vi "Copy.vi"(8 "error in (no error)":errorcluster, 10 "NT Base in":refnum<class "NT Base.lvclass">, 11 "NT Base in":refnum<class "NT Base.lvclass">) -> (0 "error out":errorcluster, 3 "NT Base out":refnum<class "NT Base.lvclass">)   [LabVIEW 2020, in "PV Access.lvlib" / "PV Data.lvlib" / "NT Base.lvclass"]
uses:
  NT Base.lvclass
  NT Base.lvclass/NT Base.ctl
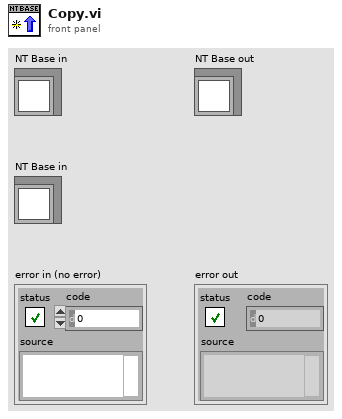
[diagram p1: front panel]
types:
  T1 = typedef "PV Access.lvlib/PV Data.lvlib/Type Code.ctl" = enum8{"Null", "Bool", "BoolA", "Int8", "Int8A", "Int16", "Int16A", "Int32", "Int32A", "Int64", "Int64A", "UInt8", "UInt8A", "UInt16", "UInt16A", "UInt32", "UInt32A", "UInt64", "UInt64A", "Float32", "Float32A", "Float64", "Float64A", "String", "StringA", "Struct", "StructA", "Union", "UnionA", "Any", "AnyA"}
  T2 = typedef "PV Access.lvlib/PV Data.lvlib/Timestamp.ctl" = cluster{"Timestamp":timestamp, "User Tag":i32}
  T3 = typedef "PV Access.lvlib/PV Data.lvlib/Alarm.ctl" = cluster{"Severity":T4, "Status":T5, "Message":string}
  T4 = typedef "PV Access.lvlib/PV Data.lvlib/Alarm Severity.ctl" = enum32{"no", "minor", "major", "record", "invalid", "undefined", ""}
  T5 = typedef "PV Access.lvlib/PV Data.lvlib/Alarm Status.ctl" = enum32{"no", "device", "driver", "record", "db", "conf", "undefined", "client"}
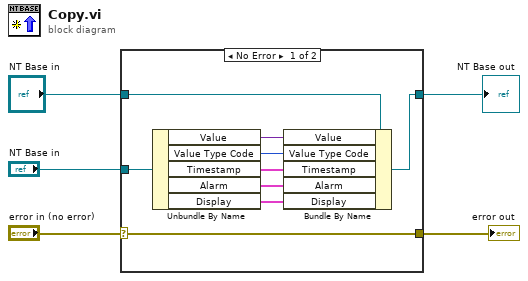
[diagram p0: block diagram]
diagram:
  n1 = case shown="No Error" "error in (no error)" {
    selector: "error in (no error)" -> [w14 w16]
    tunnel: [w14 w16] -> w4
    tunnel: [w6 w15] -> w2
    tunnel: "NT Base in" -> [w12 w15]
    tunnel: "NT Base in" -> [w13 _]
    frame No Error {
      n2 = Unbundle By Name(w13) -> ("Value"=w11:variant, "Value Type Code"=w10:T1, "Timestamp"=w9:T2, "Alarm"=w8:T3, "Display"=w7:cluster{"Description":string})
      n3 = Bundle By Name(cluster=w12, "Value"=w11, "Value Type Code"=w10, "Timestamp"=w9, "Alarm"=w8, "Display"=w7) -> (w6:refnum<class "NT Base.lvclass">)
    }
    frame Error {
    }
  }
  "error out" <- w4
  "NT Base out" <- w2
